vi "Save data.vi"(8 "error in (no error)":errorcluster, 10 "signal out":waveform(dbl), 11 "Logging Tdms in":refnum<class "Logging Tdms.lvclass">) -> (0 "error out":errorcluster, 3 "Logging Txt out":refnum<class "Logging Txt.lvclass">)   [LabVIEW 2020, in "Logging Tdms.lvlib" / "Logging Tdms.lvclass"]
uses:
  Logging Tdms.lvclass
  C:/Users/Alex/Documents/Tarea-Actor/Logging Txt/Logging Txt/Logging Txt.lvclass
  Logging Txt/Logging Txt/Logging Txt.lvclass
  Logging Txt/Logging Txt/Logging Txt.lvclass/Logging Txt.ctl
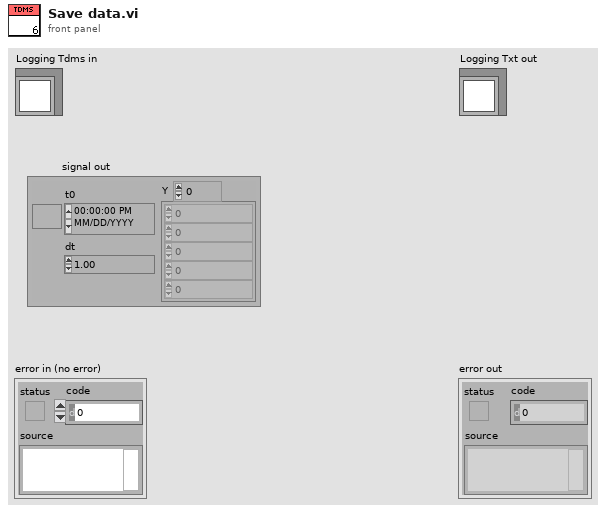
[diagram p1: front panel]
types:
  T1 = enum16{"open", "open or create", "create or replace", "create", "open (read-only)"}
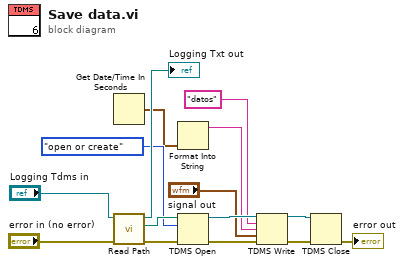
[diagram p0: block diagram]
diagram:
  n1 = Get Date/Time In Seconds() -> (seconds since 1Jan1904=w1:timestamp)
  n2 = call "Read Path.vi"("error in (no error)"="error in (no error)", "Logging Txt in"="Logging Tdms in") -> ("error out"=w6:errorcluster, "Path"=w14:path, "Logging Txt out"=→"Logging Txt out":refnum<class "Logging Tdms.lvclass">)  [unwired: 7 in]
  n3 = Format Into String(w1) -> (resulting string=w2:string)  [unwired: 3 in, 1 out]
  n4 = TDMS Open(8:w6, 10:T1."open or create" ("operation (0:open)"), 11:w14) -> (0:w10:errorcluster, 3:w12:refnum<k34>)  [unwired: 4 in]
  n5 = TDMS Write(0:w12, 5:"datos" ("group name in (Untitled)"), 7:w2, 9:"signal out", 11:w10) -> (4:w11:refnum<k34>, 15:w9:errorcluster)  [unwired: 1 in, 2 out]
  n6 = TDMS Close(8:w9, 11:w11) -> (0:→"error out":errorcluster)  [unwired: 1 out]
